vi "GetDataForExcel.CalcMean.vi"(1 "Input Array":dbl[][](array[numeric])) -> (0 "Array":dbl[](array[numeric]))   [LabVIEW 2013, in "main.lvlib"]
uses:
  main.lvlib
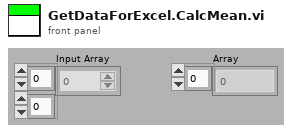
[diagram p1: front panel]
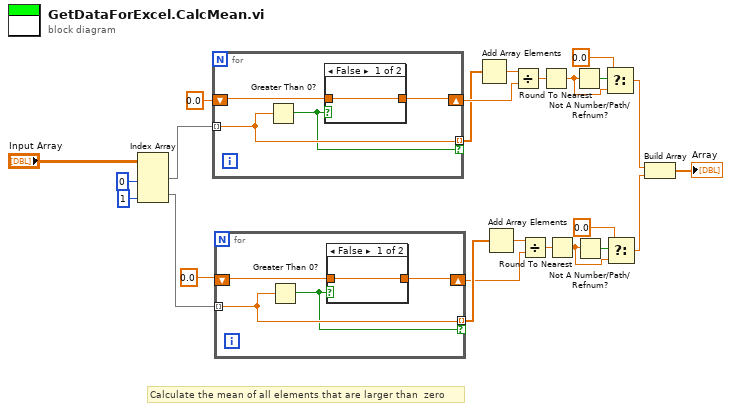
[diagram p0: block diagram]
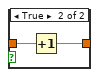
[diagram p2: hidden frame]
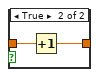
[diagram p3: hidden frame]
diagram:
  # "Calculate the mean of all elements that are larger than  zero"
  n1 = Index Array(array="Input Array", index (col) #1=0 ("disabled index (col)"), index (col) #2=1 ("disabled index (col)")) -> (element #1=w14:dbl[], element #2=w3:dbl[])  [unwired: 2 in]
  n2 = for {
    shift-right: [w28] -> w16
    shift-left: 0.0 -> [w27]
    tunnel: w14 -> [w26] mode=indexing
    tunnel: [w26] -> w5 mode=indexing if=w25
    n3 = Greater Than 0?(x=w26) -> (x > 0?=w25:bool)
    n4 = case shown="False" w25 {
      tunnel: [w29 w31] -> w28
      tunnel: w27 -> [w29 w30]
      frame False {
      }
      frame True {
        n5 = Increment(x=w30) -> (x+1=w31:dbl)
      }
    }
  }
  n6 = for {
    shift-right: [w35] -> w1
    shift-left: 0.0 -> [w34]
    tunnel: w3 -> [w33] mode=indexing
    tunnel: [w33] -> w2 mode=indexing if=w32
    n7 = Greater Than 0?(x=w33) -> (x > 0?=w32:bool)
    n8 = case shown="False" w32 {
      tunnel: [w36 w38] -> w35
      tunnel: w34 -> [w36 w37]
      frame False {
      }
      frame True {
        n9 = Increment(x=w37) -> (x+1=w38:dbl)
      }
    }
  }
  n10 = Add Array Elements(numeric array=w5) -> (sum=w18:dbl)
  n11 = Add Array Elements(numeric array=w2) -> (sum=w19:dbl)
  n12 = Divide(x=w18, y=w16) -> (x/y=w23:dbl)
  n13 = Divide(x=w19, y=w1) -> (x/y=w24:dbl)
  n14 = Round To Nearest(number=w23) -> (nearest integer value=w7:dbl)
  n15 = Round To Nearest(number=w24) -> (nearest integer value=w12:dbl)
  n16 = Not A Number/Path/Refnum?(number/path/refnum=w7) -> (NaN/Path/Refnum?=w9:bool)
  n17 = Not A Number/Path/Refnum?(number/path/refnum=w12) -> (NaN/Path/Refnum?=w13:bool)
  n18 = Select(t=0.0, s=w9, f=w7) -> (s? t:f=w6:dbl)
  n19 = Select(t=0.0, s=w13, f=w12) -> (s? t:f=w10:dbl)
  n20 = Build Array(w6, w10) -> (→"Array":dbl[])
